vi "Teepee.vi"(10 "Coefficient":dbl=1.0, 11 "Actual":dbl) -> (3 "Teepee-ed":dbl)   [LabVIEW 2013]
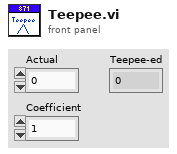
[diagram p1: front panel]
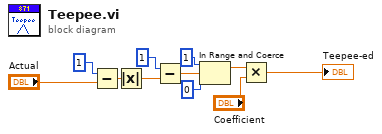
[diagram p0: block diagram]
diagram:
  n1 = Subtract(x=1, y="Actual") -> (x-y=w11:dbl)
  n2 = Absolute Value(x=w11) -> (abs(x)=w10:dbl)
  n3 = Subtract(x=1, y=w10) -> (x-y=w8:dbl)
  n4 = In Range and Coerce(upper limit=1, x=w8, lower limit=0) -> (coerced(x)=w3:dbl)  [unwired: 1 out]
  n5 = Multiply(x=w3, y="Coefficient") -> (x*y=→"Teepee-ed":dbl)
